vi "New String Handler.vi"(8 "auto-scroll? (T)":bool=TRUE, 9 "multi-line? (T)":bool=TRUE, 10 "formatter (format string)":refnum<class "Formatter.lvclass">, 11 "string control":refnum<vi>) -> (3 "new string handler":refnum<class "String Handler.lvclass">)   [LabVIEW 2018, in "GLog.lvlib" / "String Handler.lvclass"]
uses:
  String Handler.lvclass
  C:/Users/Colin/Documents/software_projects/glog/src/api/extension/formatting_handler_interface/Formatting Handler.lvclass
  extension/formatter_interface/Formatter.lvclass
  String Handler.lvclass/String Handler.ctl
  extension/formatting_handler_interface/Formatting Handler.lvclass/Formatting Handler.ctl
  e16c3569-761e-436c-a097-92f193021b46.vi
  formatters/format_string_formatter/Format String.lvclass
  C:/Users/Colin/Documents/software_projects/glog/src/api/extension/formatter_interface/Formatter.lvclass
  <vilib>/Utility/LVClass/Get LV Class Name.vi
  <vilib>/Utility/LVClass/Get LV Class Default Value By Name.vi
  extension/formatting_handler_interface/Formatting Handler.lvclass
panel:
  # "Connector Pane"
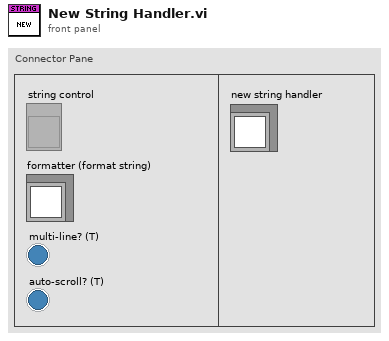
[diagram p1: front panel]
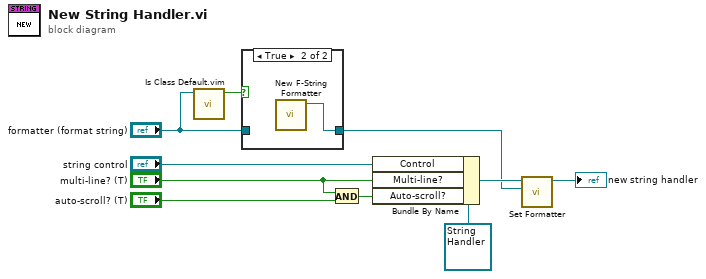
[diagram p0: block diagram]
diagram:
  n1 = call "Is Class Default.vim"("class"="formatter (format string)") -> ("is default?"=w7:bool)  [unwired: 9 in, 1 out]
  n2 = case shown="True" w7 {
    tunnel: "formatter (format string)" -> [w11 _]
    tunnel: [w11 w12] -> w1
    frame False {
    }
    frame True {
      n3 = call "New F-String Formatter.vi"() -> ("new f-string formatter"=w12:refnum<class "Format String.lvclass">)  [unwired: 11 in]
    }
  }
  n4 = And(x="multi-line? (T)", y="auto-scroll? (T)") -> (x .and. y?=w3:bool)
  n5 = Bundle By Name(cluster=refnum<class "String Handler.lvclass"> refnum ("new string handler"), "Control"="string control", "Multi-line?"="multi-line? (T)", "Auto-scroll?"=w3) -> (w9:refnum<class "String Handler.lvclass">)
  n6 = call "Set Formatter.vi"("formatter"=w1, "handler in"=w9) -> ("handler out"=→"new string handler":refnum<class "String Handler.lvclass">)  [unwired: 9 in]
